vi "RabiFlop1762WithPumpingHWT2.vi"() -> ()   [LabVIEW 2012]
uses:
  <vilib>/Utility/file.llb/Write To Spreadsheet File (DBL).vi
panel:
  in  "Cooling Delay?":bool
  in  "Cooling Delay(ms)":u32
  in  "Heat Time(units of 1 us)":dbl
  in  "End (us)":dbl=200.0
  in  "Step (us)":dbl=10.0
  out "Current Time (us)":dbl=210.0
  in  "Start (us)":dbl
  in  "Frequency (MHz)":dbl=83.847
  out "digital waveform out 3":digitalwaveform(waveform)={"t0"=timestamp(0 s since 1904-01-01), "dt"=1e-07, "Y"={"transitions"=[0, 2100, 2200, 2300, 2301, 2501, 2601], "data"=[[1, 1, 1, 0, 0], [1, 0, 1, 0, 0], [1, 0, 0, 0, 0], [0, 0, 0, 0, 0], [0, 0, 0, 0, 1], [0, 0, 0, 0, 0], [0, 1, 1, 0, 0]]}, "error"={"status"=FALSE, "code"=37421928, "source"=""}}
  out "10xwindow":i32
  out "10xdiscr":dbl
  out "DARK?":i32(graph)=50
  out "Counts":i32=50
  out "DARK?":bool
  out "PMT Counts":i32(graph)=10
  in  "PMT sample time":dbl=0.05
  out "Counts after 1762":i32=10
  out "OuterLoop":i32=20
  out "InnerLoop":i32=99
  out "Bright Events":dbl
  in  "Discriminator Level\n (Bright/Dark)":i32=28
  out "digital waveform out 2":digitalwaveform(waveform)={"t0"=timestamp(0 s since 1904-01-01), "dt"=1e-07, "Y"={"transitions"=[0, 2100, 2200, 2300, 2301, 2511, 2611], "data"=[[1, 1, 1, 0, 0], [1, 0, 1, 0, 0], [1, 0, 0, 0, 0], [0, 0, 0, 0, 0], [0, 0, 0, 0, 1], [0, 0, 0, 0, 0], [0, 1, 1, 0, 0]]}, "error"={"status"=FALSE, "code"=37421928, "source"=""}}
  in  "Comment":string="SPAOM, DPAOM = 90 MHz"
  in  "B Field":dbl=2.26
  in  "RF Power":dbl
  out "Counts finding bright ion":dbl=50.0
  in  "BG Cutoff Limit":dbl=45.0
  in  "Runs per data point":dbl=100.0
  out "Path":path=path "c:/data/1762 Scans/2014-06-19_17-15-54_1762scanWithPumping.txt"
  out "Frequency Scan":cluster{dbl, dbl}[](graph)=[{0.0, 1.03}, {10.0, 0.99}, {20.0, 0.9}, {30.0, 0.74}, {40.0, 0.68}, {50.0, 0.63}, {60.0, 0.67}, {70.0, 0.51}, {80.0, 0.69}, {90.0, 0.64}, {100.0, 0.6}, {110.0, 0.7}, {120.0, 0.63}, {130.0, 0.61}, {140.0, 0.61}, {150.0, 0.54}, {160.0, 0.65}, {170.0, 0.62}, {180.0, 0.59}, {190.0, 0.61}, {200.0, 0.67}]
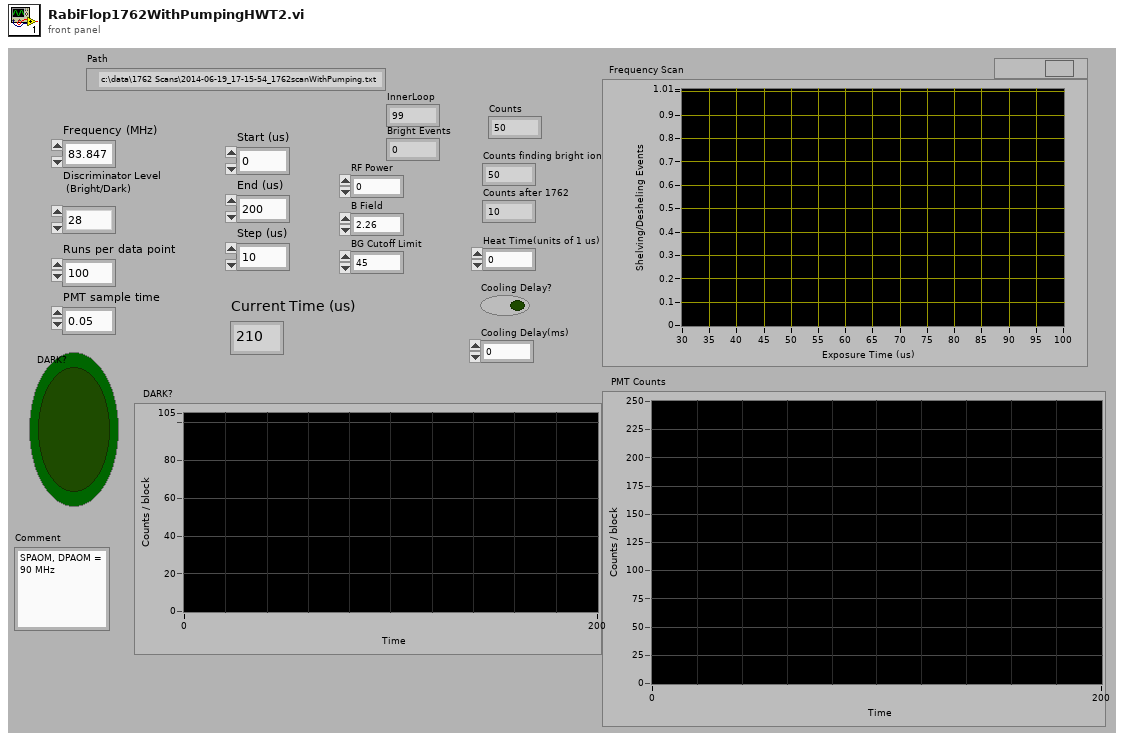
[diagram p1: front panel]
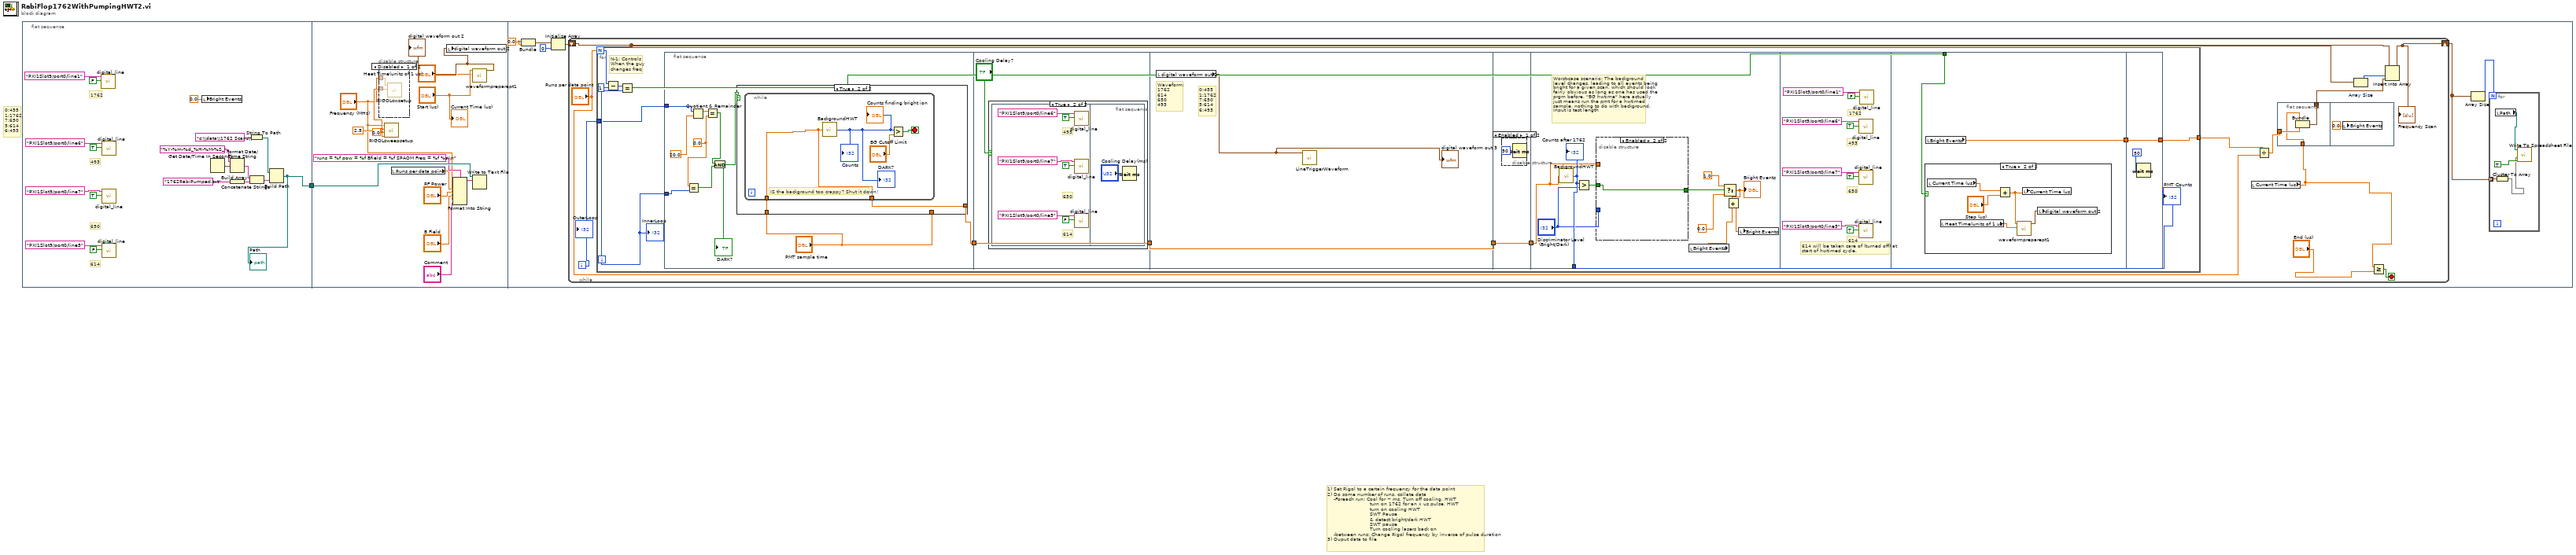
[diagram p0: block diagram]
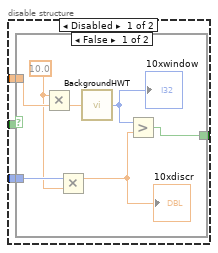
[diagram p6: hidden frame]
diagram:
  # "0:455\n1:1762\n7:650\n5:614\n6:493"
  # "1) Set Rigol to a certain frequency for the data point\n2) Do some number of runs, collate data\n    -Foreach run: Cool for ~ ms, Turn off cooling, HWT\n                           turn on 1762 for an x us pulse, HWT\n                           turn on cooling HWT\n                           SWT Pause\n                           & detect bright/dark HWT\n                           SWT pause\n                           Turn cooling lasers back on \n    -between runs: Change Rigol frequency by inverse of pulse duration\n3) Ouput data to file"
  n1 = flat-sequence {
    tunnel: [w11] -> w1
    tunnel: w1 -> [w32]
    frame #0 {
      # "614"
      # "650"
      # "493"
      # "1762"
      n2 = call "digital_line.vi"("Boolean"=FALSE, "lines"=tag "PXI1Slot9/port0/line1") -> ()  [unwired: 5 in, 1 out]
      n3 = call "digital_line.vi"("Boolean"=TRUE, "lines"=tag "PXI1Slot9/port0/line6") -> ()  [unwired: 5 in, 1 out]
      n4 = call "digital_line.vi"("Boolean"=TRUE, "lines"=tag "PXI1Slot9/port0/line7") -> ()  [unwired: 5 in, 1 out]
      n5 = call "digital_line.vi"("Boolean"=FALSE, "lines"=tag "PXI1Slot9/port0/line5") -> ()  [unwired: 5 in, 1 out]
      n6 = local write "Bright Events"(0.0 ("Bright Events")) -> ()
      n7 = Get Date/Time In Seconds() -> (seconds since 1Jan1904=w13:timestamp)
      n8 = Format Date/Time String(time format string (%c)="%Y-%m-%d_%H-%M-%S_", seconds (now)=w13) -> (date/time string=w15:string)  [unwired: 1 in]
      n9 = Build Array("1762RabiPumped.txt") -> (w18:string[])
      n10 = String To Path(string="c:\\data\\1762 Scans\\") -> (path=w19:path)
      n11 = Concatenate Strings(w15, w18) -> (w17:string)
      n12 = Build Path(base path=w19, name or relative path=w17) -> (appended path=w11:path)
      "Path" <- w11
    }
    frame #1 {
      w23 = 0.0 ("Time (ms)")
      w24 = 2.5 ("Amplitude (Vpp)")
      n13 = disable-structure shown="Disabled" {
        disable-tunnel: w24 -> [w34 _]
        disable-tunnel: "Frequency (MHz)" -> [w33 _]
        frame Disabled {
          n14 = call "RIGOLcwsetup.vi"("Amplitude (Vpp)"=w34, "Frequency (MHz)"=w33) -> ()  [unwired: 10 in]
        }
        frame Enabled {
        }
      }
      n15 = call "RIGOLsweepsetup.vi"("AP Sweep Width (MHz)"=w23, "Time (ms)"=w23, "Amplitude (Vpp)"=w24, "Frequency (MHz)"="Frequency (MHz)") -> ()  [unwired: 8 in]
      n16 = local read "Runs per data point"() -> (w29:dbl)
      n17 = Format Into String(format string="runs = %f pow = %f Bfield = %f SPAOM Freq = %f %s\\n", w29, "RF Power", "B Field", "Frequency (MHz)", "Comment") -> (resulting string=w30:string)  [unwired: 2 in, 1 out]
      n18 = call "waveformpreparept1.vi"("Heat Time(units of 1 us)"="Heat Time(units of 1 us)", "1762 pulse length (units of 1 us)"="Start (us)") -> ("digital waveform out 2"=w26:digitalwaveform)  [unwired: 7 in]
      "digital waveform out 2" <- w26
      n19 = local write "digital waveform out 2"(w26) -> ()
      n20 = Write to Text File(file (use dialog)=w32, text=w30) -> ()  [unwired: 2 in, 3 out]
      "Current Time (us)" <- "Start (us)"
    }
    frame #2 {
      w39 = 0.0
      n21 = Bundle(w39, w39) -> (w40:cluster{dbl, dbl})  [unwired: 1 in]
      n22 = Initialize Array(w40, 0) -> (w37:cluster{dbl, dbl}[])
      n23 = while {
        shift-right: [w52] -> w35
        shift-left: w37 -> [w53]
        i -> [w51]
        stop <- w55 stop-if-true
        n24 = for {
          N: "Runs per data point" -> [w69]
          tunnel: [w68] -> w49
          tunnel: w51 -> [w65]
          i -> [w66]
          # "N-1: Controls\nWhen the guy\nchanges freq"
          n25 = Subtract(x=w69, y=1) -> (x-y=w72:i32)
          n26 = Equal?(x=w72, y=w66) -> (x = y?=w70:bool)
          n27 = flat-sequence {
            tunnel: w66 -> [w80]
            tunnel: w65 -> [w75]
            tunnel: [w74] -> w61
            tunnel: w61 -> [w91]
            tunnel: [w91] -> w60
            tunnel: [w100] -> w62
            tunnel: w60 -> [w100]
            tunnel: [w101] -> w63
            tunnel: w62 -> [w101]
            tunnel: w63 -> [w105]
            tunnel: [w107] -> w64
            tunnel: w70 -> [w134]
            tunnel: [w135] -> w67
            tunnel: [w142] -> w68
            tunnel: w67 -> [w142]
            frame #0 {
              w79 = 0.0 ("x")
              n28 = Equal?(x=w79, y=w80) -> (x = y?=w77:bool)
              n29 = Quotient & Remainder(x=w75, y=20.0 ("Rerun BG Every\nnth freq point")) -> (x-y*floor(x/y)=w81:dbl)  [unwired: 1 out]
              n30 = Equal?(x=w81, y=w79) -> (x = y?=w78:bool)
              n31 = And(x=w78, y=w77) -> (x .and. y?=w76:bool)
              "DARK?" <- w76
              n32 = case shown="True" w76 {
                tunnel: [w83 w85] -> w74
                tunnel: "PMT sample time" -> [w83 _]
                tunnel: "PMT sample time" -> [_ w84]
                frame False {
                }
                frame True {
                  n33 = while {
                    tunnel: [w86] -> w85
                    tunnel: w84 -> [w86]
                    stop <- w88 stop-if-true
                    # "IS the background too crappy? Shut it down!"
                    n34 = call "BackgroundHWT.vi"("Sample Time(seconds)"=w86) -> ("Counts"=w87:i32)
                    "Counts finding bright ion" <- w87
                    "Counts" <- w87
                    "DARK?" <- w87
                    n35 = Greater?(x=w87, y="BG Cutoff Limit") -> (0:w88:bool)
                  }
                }
              }
            }
            frame #1 {
              n36 = case shown="True" "Cooling Delay?" {
                frame False {
                }
                frame True {
                  n37 = flat-sequence {
                    frame #0 {
                      # "614"
                      # "650"
                      # "493"
                      n38 = call "digital_line.vi"("Boolean"=TRUE, "lines"=tag "PXI1Slot9/port0/line6") -> ()  [unwired: 5 in, 1 out]
                      n39 = call "digital_line.vi"("Boolean"=TRUE, "lines"=tag "PXI1Slot9/port0/line7") -> ()  [unwired: 5 in, 1 out]
                      n40 = call "digital_line.vi"("Boolean"=FALSE, "lines"=tag "PXI1Slot9/port0/line5") -> ()  [unwired: 5 in, 1 out]
                    }
                    frame #1 {
                      n41 = Wait (ms)(milliseconds to wait="Cooling Delay(ms)") -> ()  [unwired: 1 out]
                    }
                  }
                }
              }
            }
            frame #2 {
              # "0:455\n1:1762\n7:650\n5:614\n6:493"
              # "Waveform:\n1762\n614\n650\n493"
              n42 = local read "digital waveform out 2"() -> (w99:digitalwaveform)
              "digital waveform out 3" <- w99
              n43 = call "LineTriggerWaveform.vi"("digital waveform in"=w99) -> ()  [unwired: 11 in]
            }
            frame #3 {
              n44 = disable-structure shown="Enabled" {
                frame Enabled {
                  n45 = Wait (ms)(milliseconds to wait=u32 50) -> ()  [unwired: 1 out]
                }
                frame Disabled {
                }
              }
            }
            frame #4 {
              # "Worst-case scenario: The background\nlevel changes, leading to all events being\nbright for a given scan, which should look\nfairly obvious as long as one has used the\nprgm before. \"BG hwtime\" here actually\njust means run the pmt for a hwtimed\nsample, nothing to do with background.\nInput is test length"
              n46 = call "BackgroundHWT.vi"("Sample Time(seconds)"=w105) -> ("Counts"=w107:i32)
              "Counts after 1762" <- w107
              n47 = Greater?(x=w107, y="Discriminator Level\n (Bright/Dark)") -> (0:w106:bool)
              n48 = disable-structure shown="Enabled" {
                disable-tunnel: w106 -> [w116 w125]
                disable-tunnel: [w115 w125] -> w103
                disable-tunnel: w105 -> [w114 _]
                disable-tunnel: "Discriminator Level\n (Bright/Dark)" -> [w113 _]
                frame Disabled {
                  n49 = case shown="False" w116 {
                    selector: w116 -> [_ w124]
                    tunnel: [w119 w124] -> w115
                    tunnel: w114 -> [w123 _]
                    tunnel: w113 -> [w120 _]
                    frame False {
                      w117 = 10.0 ("x")
                      n50 = Multiply(x=w117, y=w123) -> (x*y=w122:dbl)
                      n51 = Multiply(x=w120, y=w117) -> (x*y=w118:dbl)
                      "10xdiscr" <- w118
                      n52 = call "BackgroundHWT.vi"("Sample Time(seconds)"=w122) -> ("Counts"=w121:i32)
                      "10xwindow" <- w121
                      n53 = Greater?(x=w121, y=w118) -> (0:w119:bool)
                    }
                    frame True {
                    }
                  }
                }
                frame Enabled {
                }
              }
              n54 = local read "Bright Events"() -> (w108:dbl)
              n55 = Select(t=1.0, s=w103, f=0.0) -> (s? t:f=w110:dbl)
              "Bright Events" <- w110
              n56 = Add(x=w110, y=w108) -> (x+y=w109:dbl)
              n57 = local write "Bright Events"(w109) -> ()
            }
            frame #5 {
              # "614 will be taken care of (turned off) at\nstart of hwtimed cycle."
              # "614"
              # "650"
              # "493"
              # "1762"
              n58 = call "digital_line.vi"("Boolean"=TRUE, "lines"=tag "PXI1Slot9/port0/line6") -> ()  [unwired: 5 in, 1 out]
              n59 = call "digital_line.vi"("Boolean"=TRUE, "lines"=tag "PXI1Slot9/port0/line7") -> ()  [unwired: 5 in, 1 out]
              n60 = call "digital_line.vi"("Boolean"=TRUE, "lines"=tag "PXI1Slot9/port0/line5") -> ()  [unwired: 5 in, 1 out]
              n61 = call "digital_line.vi"("Boolean"=FALSE, "lines"=tag "PXI1Slot9/port0/line1") -> ()  [unwired: 5 in, 1 out]
            }
            frame #6 {
              n62 = case shown="True" w134 {
                frame False {
                }
                frame True {
                  n63 = local read "Current Time (us)"() -> (w140:dbl)
                  n64 = local read "Heat Time(units of 1 us)"() -> (w136:dbl)
                  n65 = Add(x=w140, y="Step (us)") -> (x+y=w138:dbl)
                  n66 = call "waveformpreparept1.vi"("Heat Time(units of 1 us)"=w136, "1762 pulse length (units of 1 us)"=w138) -> ("digital waveform out 2"=w137:digitalwaveform)  [unwired: 7 in]
                  n67 = local write "Current Time (us)"(w138) -> ()
                  n68 = local write "digital waveform out 2"(w137) -> ()
                }
              }
              n69 = local read "Bright Events"() -> (w135:dbl)
            }
            frame #7 {
              n70 = Wait (ms)(milliseconds to wait=u32 50) -> ()  [unwired: 1 out]
            }
          }
          "InnerLoop" <- w66
          "PMT Counts" <- w64
        }
        n71 = local read "Current Time (us)"() -> (w46:dbl)
        n72 = Divide(x=w49, y="Runs per data point") -> (x/y=w48:dbl)
        n73 = flat-sequence {
          tunnel: w48 -> [w58]
          tunnel: [w57] -> w50
          tunnel: w46 -> [w56]
          frame #0 {
            n74 = Bundle("Current Time (us)"=w56, w58) -> (w57:cluster{"Current Time (us)":dbl, dbl})  [unwired: 1 in]
          }
          frame #1 {
            n75 = local write "Bright Events"(0.0 ("Bright Events")) -> ()
          }
        }
        n76 = Array Size(array=w53) -> (size(s)=w54:i32)
        n77 = Greater Or Equal?(x=w46, y="End (us)") -> (x >= y?=w55:bool)
        n78 = Insert Into Array(array=w53, index=w54, new element=w50) -> (w52:cluster{dbl, dbl}[])
        "Frequency Scan" <- w52
        "OuterLoop" <- w51
      }
      n79 = Array Size(array=w35) -> (size(s)=w36:i32)
      n80 = for {
        N: w36 -> [_]
        tunnel: w35 -> [w44] mode=indexing
        n81 = local read "Path"() -> (w41:path)
        n82 = Cluster To Array(cluster=w44) -> (array=w42:dbl[])
        n83 = call-poly <vilib>:"Write To Spreadsheet File.vi"("append to file? (new file:F)"=TRUE, "1D data"=w42, "file path (dialog if empty)"=w41) -> ()  [unwired: 5 in, 1 out]
      }
    }
  }
